vi "Arrange Diagram.vi"(8 "error in (no error)":errorcluster, 10 "Shift?":bool, 11 "VI Refnum in":refnum<vi>) -> (0 "error out":errorcluster, 3 "VI Refnum out":refnum<vi>)   [LabVIEW 2019, in "Builtins.lvlib"]
doc: "Arranges the selected diagram objects according to horizontal position and adjacent terminal location.\n\nCreated by: Ryan Pacini"
uses:
  Builtins.lvlib
  Arrange.ctl
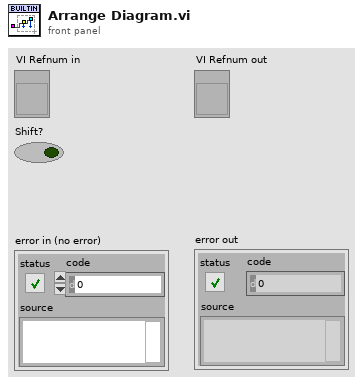
[diagram p1: front panel]
types:
  T1 = typedef "Builtins.lvlib/Arrange.ctl" = enum8{"left_to_right", "right_to_left"}
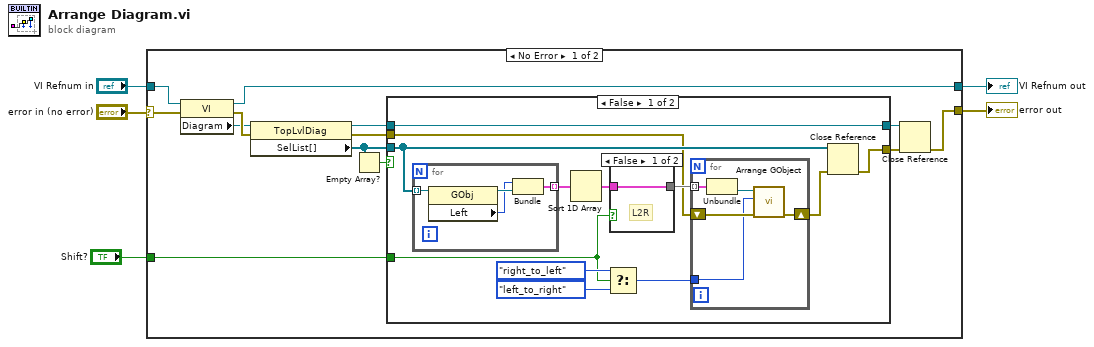
[diagram p0: block diagram]
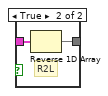
[diagram p2: hidden frame]
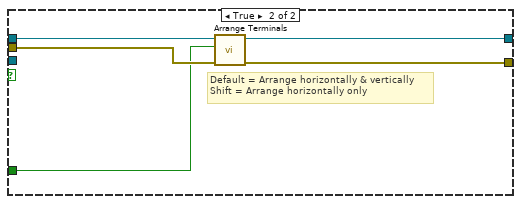
[diagram p3: hidden frame]
diagram:
  n1 = case shown="No Error" "error in (no error)" {
    selector: "error in (no error)" -> [w17 w48]
    tunnel: "VI Refnum in" -> [w18 w49]
    tunnel: [w10 w49] -> w4
    tunnel: [w6 w48] -> w2
    tunnel: "Shift?" -> [w14 _]
    frame No Error {
      n2 = property class="VI"(reference=w18, error in=w17) -> (reference out=w10:refnum<vi>, error out=w16:errorcluster, "Diagram"=w15:refnum<vi>)
      n3 = property class="TopLvlDiag"(reference=w15, error in=w16) -> (reference out=w9:refnum<vi>, error out=w11:errorcluster, "SelList[]"=w13:refnum<vi>[])
      n4 = Empty Array?(array=w13) -> (empty?=w12:bool)
      n5 = case shown="False" w12 {
        tunnel: [w27 w46] -> w7
        tunnel: w14 -> [w19 w43]
        tunnel: w11 -> [w25 w47]
        tunnel: w13 -> [w26 _]
        tunnel: w9 -> [w23 w45]
        tunnel: [w23 w44] -> w8
        frame False {
          n6 = for {
            tunnel: w26 -> [w42] mode=indexing
            tunnel: [w39] -> w30 mode=indexing
            n7 = property class="GObj"(reference=w42) -> (reference out=w41:refnum<vi>, "Left"=w40:i32)  [unwired: 1 in, 1 out]
            n8 = Bundle("Left"=w40, w41) -> (w39:cluster{"Left":i32, refnum<vi>})  [unwired: 1 in]
          }
          n9 = Sort 1D Array(array=w30) -> (sorted array=w29:cluster{"Left":i32, refnum<vi>}[])
          n10 = Select(t=Arrange."right_to_left" ("Arrange"), s=w19, f=Arrange."left_to_right" ("Arrange")) -> (s? t:f=w20:T1)
          n11 = case shown="False" w19 {
            tunnel: w29 -> [w31 w33]
            tunnel: [w31 w32] -> w28
            frame False {
              # "L2R"
            }
            frame True {
              # "R2L"
              n12 = Reverse 1D Array(array=w33) -> (reversed array=w32:cluster{"Left":i32, refnum<vi>}[])
            }
          }
          n13 = for {
            tunnel: w28 -> [w38] mode=indexing
            shift-right: [w36] -> w24
            shift-left: w25 -> [w35]
            tunnel: w20 -> [w34]
            n14 = Unbundle(w38) -> (w37:refnum<vi>)  [unwired: 1 out]
            n15 = call "Arrange GObject.vi"("error in (no error)"=w35, "Arrange"=w34, "GObject in"=w37) -> ("error out"=w36:errorcluster)  [unwired: 6 in, 2 out]
          }
          n16 = Close Reference(reference=w26, error in (no error)=w24) -> (error out=w27:errorcluster)
        }
        frame True {
          # "Default = Arrange horizontally & vertically\nShift = Arrange horizontally only"
          n17 = call "Arrange Terminals.vi"("error in (no error)"=w47, "Horizontal Only? (F)"=w43, "Diagram in"=w45) -> ("error out"=w46:errorcluster, "Diagram out"=w44:refnum<vi>)  [unwired: 7 in]
        }
      }
      n18 = Close Reference(reference=w8, error in (no error)=w7) -> (error out=w6:errorcluster)
    }
    frame Error {
    }
  }
  "VI Refnum out" <- w4
  "error out" <- w2
